vi "TextBoxLogCtrlMgr.Set Auto Scroll.vi"(7 "Auto Scroll":bool, 10 "error in (no error)":errorcluster, 11 "TextBoxLogCtrlMgr in":refnum<class "TextBoxLogCtrlMgr.lvclass">) -> (2 "error out":errorcluster, 3 "TextBoxLogCtrlMgr out":refnum<class "TextBoxLogCtrlMgr.lvclass">)   [LabVIEW 2024, in "EQMF.lvlib" / "String Utils.lvlib" / "TextBoxLogCtrlMgr.lvclass"]
uses:
  TextBoxLogCtrlMgr.lvclass
  TextBoxLogCtrlMgr.lvclass/TextBoxLogCtrlMgr.ctl
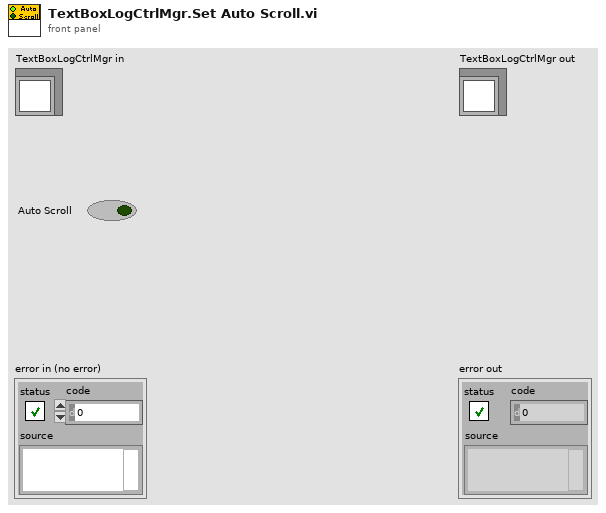
[diagram p1: front panel]
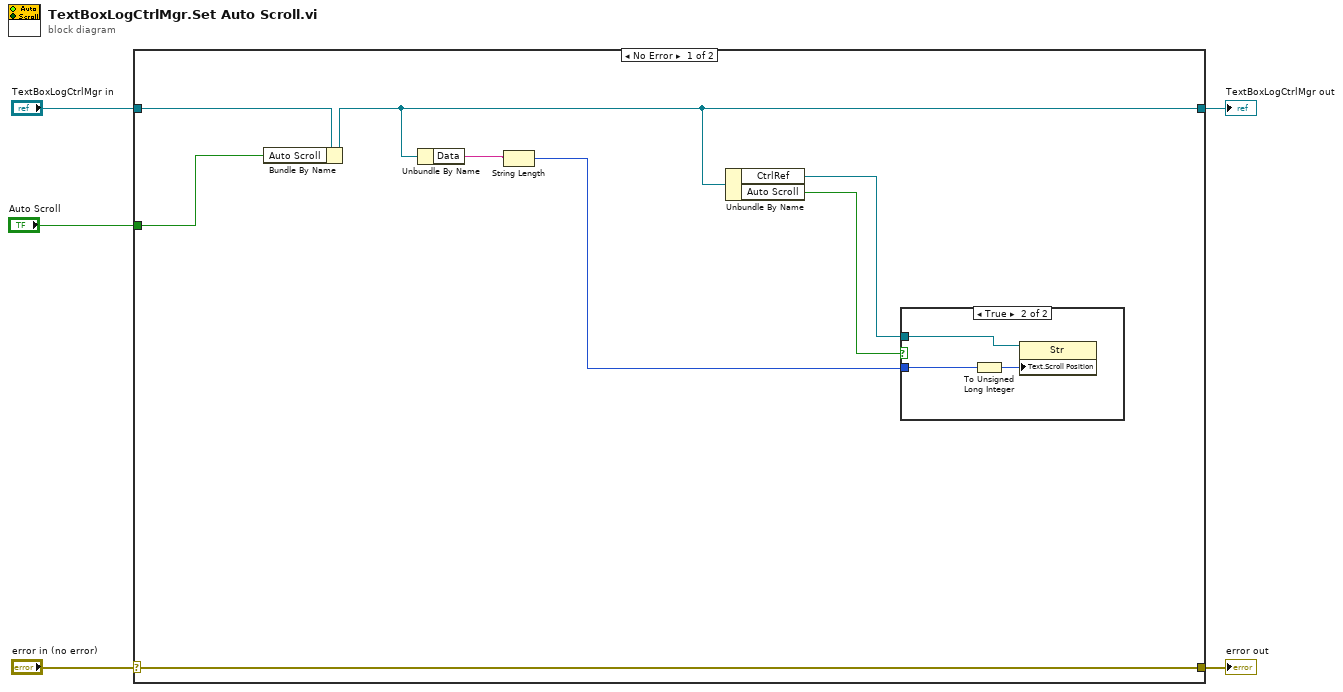
[diagram p0: block diagram]
diagram:
  n1 = case shown="No Error" "error in (no error)" {
    selector: "error in (no error)" -> [w13 w18]
    tunnel: [w13 w18] -> w4
    tunnel: [w9 w17] -> w2
    tunnel: "TextBoxLogCtrlMgr in" -> [w10 w17]
    tunnel: "Auto Scroll" -> [w8 _]
    frame No Error {
      n2 = Bundle By Name(cluster=w10, "Auto Scroll"=w8) -> (w9:refnum<class "TextBoxLogCtrlMgr.lvclass">)
      n3 = Unbundle By Name(w9) -> ("Data"=w7:string)
      n4 = String Length(string=w7) -> (length=w6:i32)
      n5 = Unbundle By Name(w9) -> ("CtrlRef"=w11:refnum<vi>, "Auto Scroll"=w12:bool)
      n6 = case shown="True" w12 {
        tunnel: w11 -> [_ w16]
        tunnel: w6 -> [_ w14]
        frame False {
        }
        frame True {
          n7 = To Unsigned Long Integer(number=w14) -> (unsigned 32bit integer=w15:u32)
          n8 = property class="Str"(reference=w16, "Text.Scroll Position"=w15) -> ()  [unwired: 1 in, 2 out]
        }
      }
    }
    frame Error {
    }
  }
  "error out" <- w4
  "TextBoxLogCtrlMgr out" <- w2
